vi "mlink_ao_scan_is_done.vi"(8 "error in (no error)":errorcluster, 11 "connection ID":i32=-1) -> (0 "error out":errorcluster, 3 "connection ID out":i32)   [LabVIEW 2009, in "MicroDAQ.lvlib" / "mlink.lvlib"]
doc: "This function checks current state of analog output scanning session."
uses:
  <instrlib>/MicroDAQ/Mlink library wraper/mlink.lvlib
  <instrlib>/MicroDAQ/MLink32.dll
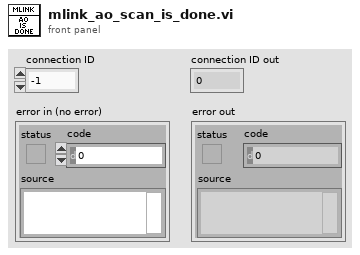
[diagram p1: front panel]
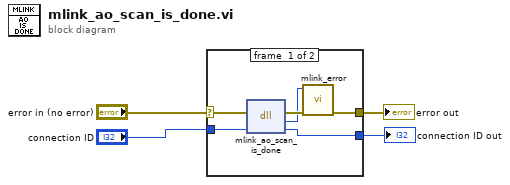
[diagram p0: block diagram]
diagram:
  n1 = case shown="No Error" "error in (no error)" {
    selector: "error in (no error)" -> [w10 w12]
    tunnel: "connection ID" -> [w9 w11]
    tunnel: [w8 w11] -> w2
    tunnel: [w5 w12] -> w1
    frame #0 {
      n2 = dll-call lib="C:/Program Files (x86)/National Instruments/LabVIEW 2009/instr.lib/MicroDAQ/MLink32.dll" fn="mlink_ao_scan_is_done" ("MLink64.dll:mlink_dsp_run")(error in=w10, "link_fd"=w9) -> (error out=w7:errorcluster, "return type"=w6:i32, "link_fd"=w8:i32)  [unwired: 2 in, 1 out]
      n3 = call <instrlib>:"mlink_error.vi"("error in (no error)"=w7, "error code"=w6) -> ("error out"=w5:errorcluster)  [unwired: 9 in]
    }
    frame #1 {
    }
  }
  "connection ID out" <- w2
  "error out" <- w1
